vi "Write path segments.vi"(8 "error in (no error)":errorcluster, 10 "Segments":string[](array[string]), 11 "URI in":refnum<class "URI.lvclass">) -> (0 "error out":errorcluster, 3 "URI out":refnum<class "URI.lvclass">)   [LabVIEW 2013, in "openURI.lvlib" / "URI.lvclass"]
uses:
  URI.lvclass
  URI.lvclass/URI.ctl
  components/path/URI-Component.Path.lvclass
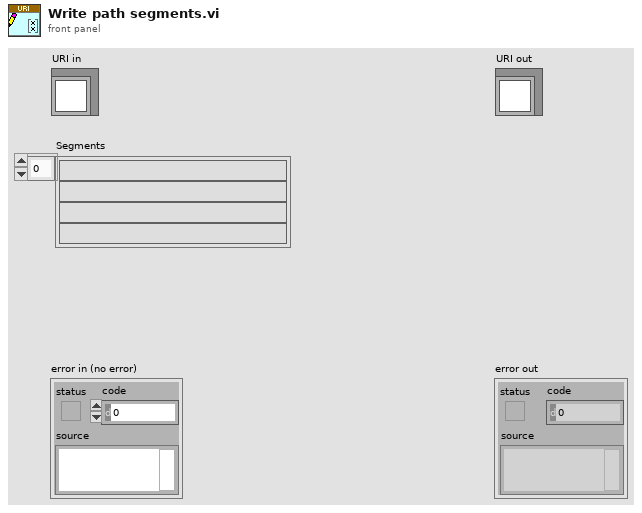
[diagram p1: front panel]
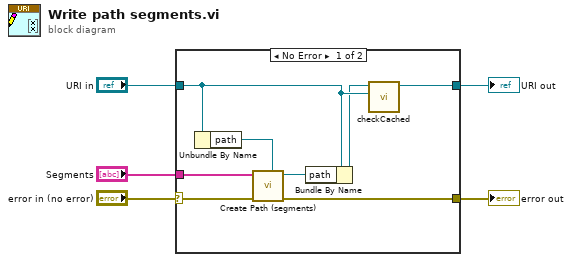
[diagram p0: block diagram]
diagram:
  n1 = case shown="No Error" "error in (no error)" {
    selector: "error in (no error)" -> [w9 w14]
    tunnel: [w12 w14] -> w4
    tunnel: [w13 w15] -> w2
    tunnel: "URI in" -> [w8 w15]
    tunnel: "Segments" -> [w11 _]
    frame No Error {
      n2 = Unbundle By Name(w8) -> ("path"=w7:refnum<class "URI-Component.Path.lvclass">)
      n3 = call "Create Path (segments).vi"("URI-Component.Path"=w7, "error in (no error)"=w9, "Segments"=w11) -> ("error out"=w12:errorcluster, "URI-Component.Path"=w10:refnum<class "URI-Component.Path.lvclass">)  [unwired: 6 in, 1 out]
      n4 = Bundle By Name(cluster=w8, "path"=w10) -> (w6:refnum<class "URI.lvclass">)
      n5 = call "checkCached.vi"("Old"=w8, "New URI"=w6) -> ("URI"=w13:refnum<class "URI.lvclass">)  [unwired: 9 in]
    }
    frame Error {
    }
  }
  "error out" <- w4
  "URI out" <- w2
